vi "ExFilterWheelOnSpect.vi"() -> ()   [LabVIEW 2010]
panel:
  out "User Name":string
  out "Serial Number":string
  out "Model Name":string
  out "Model Number":u32
  in  "?":bool
  out "Number of Filter Wheels":i16
  in  "?":bool
  out "Filter Wheel Open":bool
  out "Number Of Filters":i16=1 min=1 step=1
  in  "?":bool
  in  "?":bool
  out "Filter":i16=1 min=1 step=1
  in  "?":bool
  in  "?":bool
  in  "?":bool
  in  "Filter":i16=1 min=1 max=100 step=1
  out "error out":errorcluster
  in  "error in":errorcluster
  # "ExFilterWheelOnSpect.vi\n(Normal filter wheel via USB/COM port)\nThis example shows how access a filter wheel via a USB/COM port.\nNot all commands may be available for all filter wheels.\nNOTE: The properly configured filter wheel .ini file must be\npresent in the LabVIEW folder for filter wheel operation."
  # "This is the number of filter\nwheels setup in the .ini file."
  # "The number of filters is set in the .ini file"
  # "Note: Model Number,\nModel Name and\nSerial Number are\nobtained from the filter\nwheel.  If it does not\ncarry this information,\nthese values will be 0\nor blank.  The User\nName is taken from\nthe .ini file."
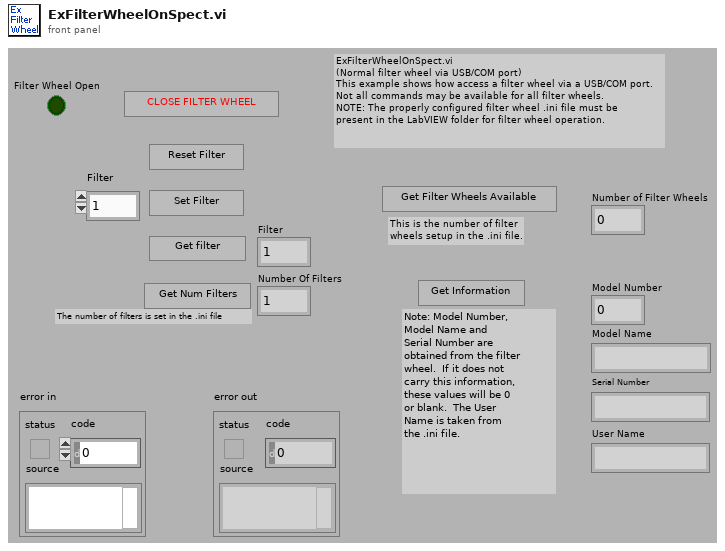
[diagram p1: front panel]
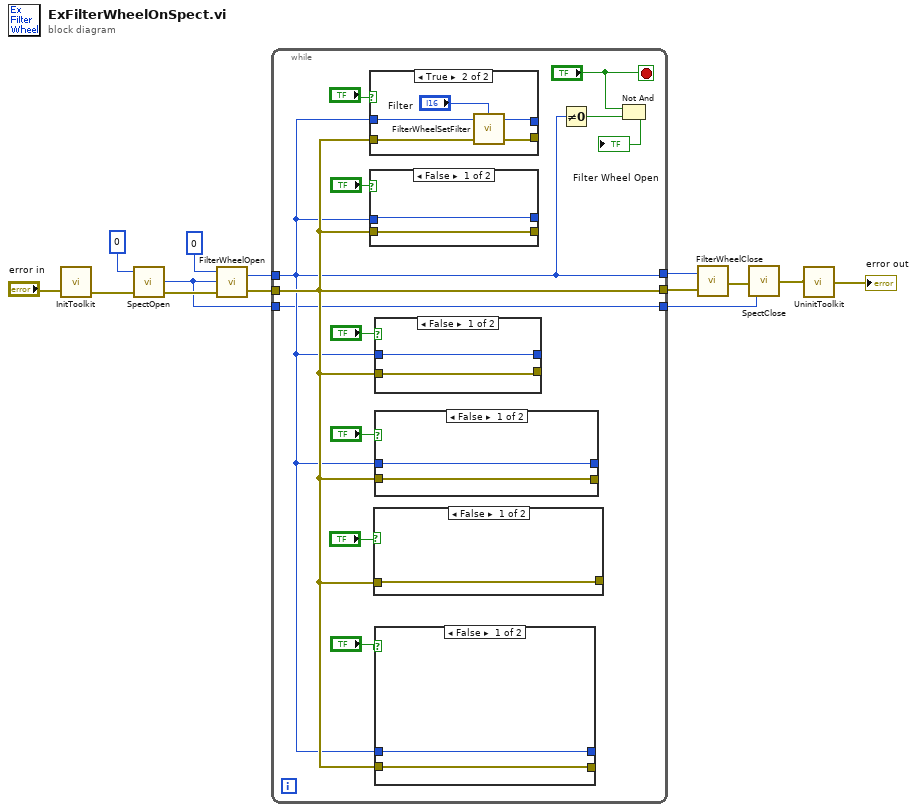
[diagram p0: block diagram]
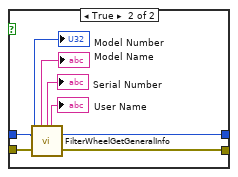
[diagram p2: hidden frame]
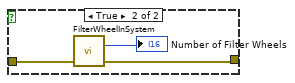
[diagram p3: hidden frame]
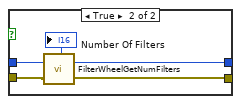
[diagram p4: hidden frame]
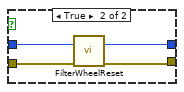
[diagram p5: hidden frame]
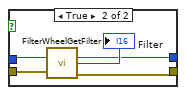
[diagram p6: hidden frame]
diagram:
  n1 = call <userlib>:"InitToolkit.vi"("error in"="error in") -> ("error out"=w8:errorcluster)
  n2 = call <userlib>:"SpectOpen.vi"("error in"=w8, "Spectrometer ID"=0) -> ("error out"=w7:errorcluster, "Spectrometer Handle"=w2:u32)  [unwired: 1 in]
  n3 = call <userlib>:"FilterWheelOpen.vi"("error in"=w7, "Device Handle"=w2, "Filter Wheel ID"=0) -> ("error out"=w12:errorcluster, "Filter Wheel Handlle"=w9:u32)
  n4 = while {
    tunnel: w9 -> [w16]
    tunnel: w12 -> [w17]
    tunnel: [w16] -> w11
    tunnel: [w17] -> w10
    tunnel: w2 -> [w15]
    tunnel: [w15] -> w1
    stop <- "?" stop-if-true
    n5 = case shown="True" "?" {
      tunnel: [w61 w67] -> _
      tunnel: [w62 w66] -> _
      tunnel: w16 -> [w62 w65]
      tunnel: w17 -> [w61 w64]
      frame False {
      }
      frame True {
        n6 = call <userlib>:"FilterWheelSetFilter.vi"("error in"=w64, "Filter"="Filter", "Filter Wheel Handle"=w65) -> ("error out"=w67:errorcluster, "Filter Wheel Handle"=w66:u32)  [unwired: 1 in]
      }
    }
    n7 = case shown="False" "?" {
      tunnel: w16 -> [w55 w60]
      tunnel: w17 -> [w54 w59]
      tunnel: [w54 w58] -> _
      tunnel: [w55 w56] -> _
      frame False {
      }
      frame True {
        n8 = call <userlib>:"FilterWheelGetFilter.vi"("error in"=w59, "Filter Wheel Handle"=w60) -> ("error out"=w58:errorcluster, "Filter Number"=→"Filter":i16, "Filter Wheel Handle"=w56:u32)  [unwired: 1 in]
      }
    }
    n9 = case shown="False" "?" {
      tunnel: w17 -> [w37 w40]
      tunnel: [w37 w39] -> _
      frame False {
      }
      frame True {
        n10 = call <userlib>:"FilterWheelInSystem.vi"("error in"=w40) -> ("Number of Filter Wheels"=→"Number of Filter Wheels":i32, "error out"=w39:errorcluster)
      }
    }
    n11 = case shown="False" "?" {
      tunnel: w17 -> [w48 w51]
      tunnel: w16 -> [w49 w53]
      tunnel: [w49 w52] -> _
      tunnel: [w48 w50] -> _
      frame False {
      }
      frame True {
        n12 = call <userlib>:"FilterWheelReset.vi"("error in"=w51, "Filter Wheel Handle"=w53) -> ("error out"=w50:errorcluster, "Filter Wheel Handle"=w52:u32)  [unwired: 1 in]
      }
    }
    n13 = case shown="False" "?" {
      tunnel: w16 -> [w42 w46]
      tunnel: [w42 w45] -> _
      tunnel: w17 -> [w41 w44]
      tunnel: [w41 w43] -> _
      frame False {
      }
      frame True {
        n14 = call <userlib>:"FilterWheelGetNumFilters.vi"("error in"=w44, "Filter Wheel Handle"=w46) -> ("error out"=w43:errorcluster, "Number of Filters"=→"Number Of Filters":i16, "Filter Wheel Handle"=w45:u32)  [unwired: 1 in]
      }
    }
    n15 = case shown="False" "?" {
      tunnel: w17 -> [w27 w31]
      tunnel: w16 -> [w28 w32]
      tunnel: [w27 w30] -> _
      tunnel: [w28 w29] -> _
      frame False {
      }
      frame True {
        n16 = call <userlib>:"FilterWheelGetGeneralInfo.vi"("Filter Wheel Handle"=w32, "error in"=w31) -> ("Model Number"=→"Model Number":u32, "User Name"=→"User Name":string, "Filter Wheel Handle"=w29:u32, "ModelName"=→"Model Name":string, "Serial Number"=→"Serial Number":string, "error out"=w30:errorcluster)
      }
    }
    n17 = Not Equal To 0?(x=w16) -> (x != 0?=w22:bool)
    n18 = Not And(1:w22, 2:"?") -> (0:→"Filter Wheel Open":bool)
  }
  n19 = call <userlib>:"FilterWheelClose.vi"("error in"=w10, "Filter Wheel Handle"=w11) -> ("error out"=w4:errorcluster)
  n20 = call <userlib>:"SpectClose.vi"("error in"=w4, "Spectrometer Handle"=w1) -> ("error out"=w3:errorcluster)
  n21 = call <userlib>:"UninitToolkit.vi"("error in"=w3) -> ("error out"=→"error out":errorcluster)
